vi "Sawtooth.vi"(0 "error in":errorcluster, 5 "Amount of Points":i32, 7 "Amplitude":dbl, 9 "DC Offset":dbl) -> (4 "error out":errorcluster, 6 "Array":dbl[](array[numeric]))   [LabVIEW 2020]
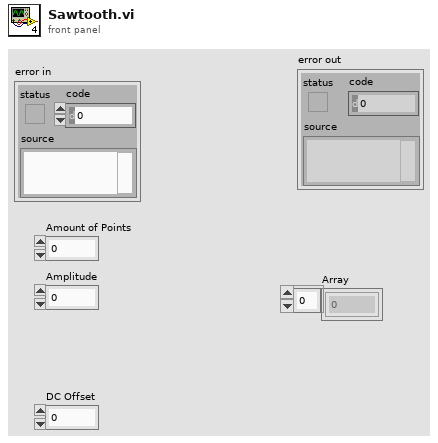
[diagram p1: front panel]
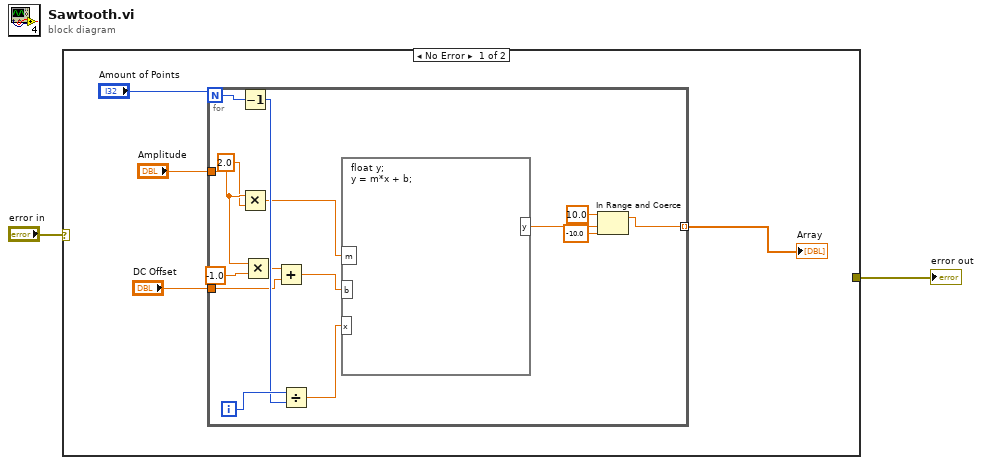
[diagram p0: block diagram]
diagram:
  n1 = case shown="No Error" "error in" {
    selector: "error in" -> [_ w22]
    tunnel: [_ w22] -> w1
    frame No Error {
      n2 = for {
        N: "Amount of Points" -> [w20]
        tunnel: "Amplitude" -> [w13]
        tunnel: "DC Offset" -> [w15]
        tunnel: [w7] -> w3 mode=indexing
        i -> [w19]
        n3 = Decrement(x=w20) -> (x-1=w18:i32)
        n4 = Multiply(x=w13, y=2.0) -> (x*y=w11:dbl)
        n5 = Multiply(x=w13, y=-1.0) -> (x*y=w16:dbl)
        n6 = Add(x=w16, y=w15) -> (x+y=w14:dbl)
        n7 = Divide(x=w19, y=w18) -> (x/y=w21:dbl)
        n8 = formula code="float y;\ny = m*x + b;"("m"=w11, "x"=w21, "b"=w14) -> ("y"=w10:dbl)
        n9 = In Range and Coerce(upper limit=10.0, x=w10, lower limit=-10.0) -> (coerced(x)=w7:dbl)  [unwired: 1 out]
      }
      "Array" <- w3
    }
    frame Error {
    }
  }
  "error out" <- w1
